vi "Get Indicator Data.vi"(6 "Connection ID":u64, 7 "Evaluate Pane Move":bool, 8 "error in (no error)":errorcluster, 9 "Values and Position":refnum<vi>[](array[refnum]), 10 "Get All":bool, 11 "Web FP In":refnum<class "Web Front Panel.lvclass">) -> (0 "error out":errorcluster, 2 "String":string, 3 "Web FP Out":refnum<class "Web Front Panel.lvclass">)   [LabVIEW 2017, in "Front Panel Publisher.lvlib" / "Web Front Panel.lvclass"]
uses:
  Web Front Panel.lvclass
  Front Panel Objects/Object_class/Object.lvclass
  Front Panel Publisher.lvlib
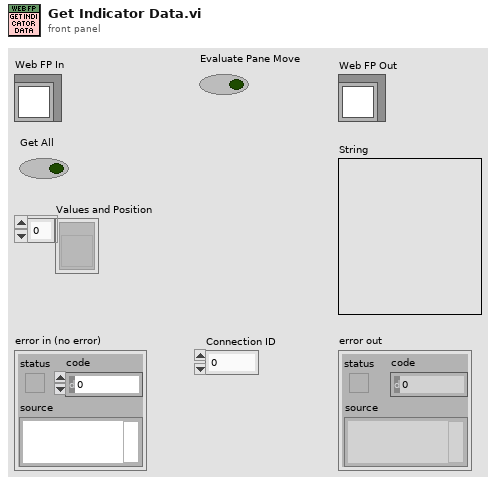
[diagram p1: front panel]
types:
  T1 = typedef "Front Panel Publisher.lvlib/Web Front Panel.lvclass/Object Attributes.ctl" = cluster{"VI Identifier":string, "VI Reference":refnum<vi>, "Controls":refnum<class "Object.lvclass">[], "Indicators":refnum<class "Object.lvclass">[], "Decorations":refnum<class "Object.lvclass">[], "VR With Previous Get":refnum<data-value>, "VR With Ring Images":refnum<data-value>}
  T2 = typedef "Front Panel Publisher.lvlib/Web Front Panel.lvclass/High Level Config Settings.ctl" = cluster{"Default Refresh Rate (ms)":i32, "Show Border":bool, "Periodic Decoration Data":bool, "Synchronous Requests":bool, "Reduce Sent Data":bool, "Recommended Control Settings":bool}
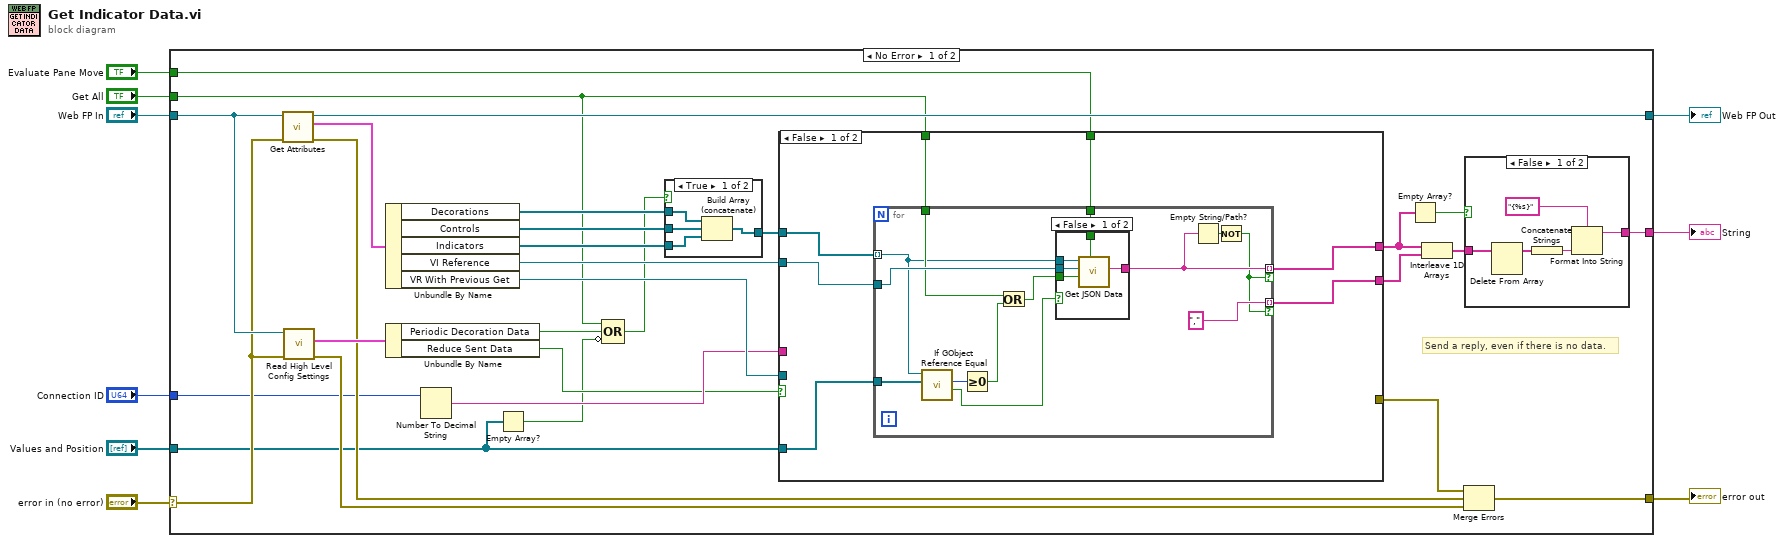
[diagram p0: block diagram]
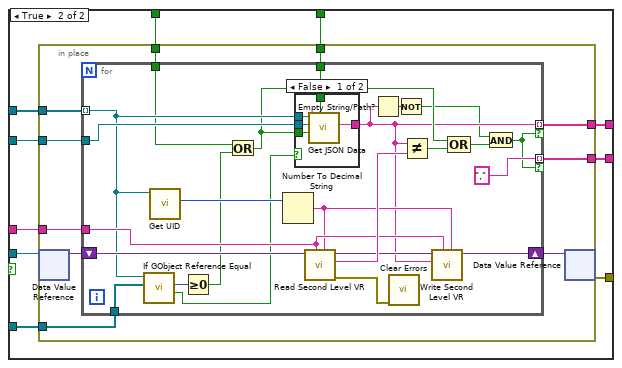
[diagram p3: hidden frame]
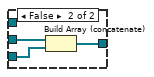
[diagram p5: hidden frame]
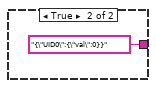
[diagram p6: hidden frame]
diagram:
  n1 = case shown="No Error" "error in (no error)" {
    selector: "error in (no error)" -> [w24 w127]
    tunnel: [w23 w127] -> w8
    tunnel: [w37 w126] -> w6
    tunnel: "Web FP In" -> [w25 w126]
    tunnel: [w33 _] -> w4
    tunnel: "Get All" -> [w14 _]
    tunnel: "Connection ID" -> [w18 _]
    tunnel: "Values and Position" -> [w15 _]
    tunnel: "Evaluate Pane Move" -> [w10 _]
    frame No Error {
      # "Send a reply, even if there is no data."
      n2 = call "Get Attributes.vi"("error in (no error)"=w24, "Web FP In"=w25) -> ("error out"=w21:errorcluster, "Data"=w38:T1, "Web FP Out"=w37:refnum<class "Web Front Panel.lvclass">)  [unwired: 6 in, 1 out]
      n3 = call "Read High Level Config Settings.vi"("error in (no error)"=w24, "Web FP In"=w25) -> ("error out"=w20:errorcluster, "High Level Config Settings"=w26:T2)  [unwired: 7 in, 1 out]
      n4 = Unbundle By Name(w38) -> ("Decorations"=w19:refnum<class "Object.lvclass">[], "Controls"=w30:refnum<class "Object.lvclass">[], "Indicators"=w32:refnum<class "Object.lvclass">[], "VI Reference"=w36:refnum<vi>, "VR With Previous Get"=w29:refnum<data-value>)
      n5 = Unbundle By Name(w26) -> ("Periodic Decoration Data"=w13:bool, "Reduce Sent Data"=w16:bool)
      n6 = Number To Decimal String(number=w18) -> (decimal integer string=w17:string)  [unwired: 1 in]
      n7 = Empty Array?(array=w15) -> (empty?=w12:bool)
      n8 = Compound Arithmetic op=OR(w14, w13, invert w12) -> (w11:bool)
      n9 = case shown="True" w11 {
        tunnel: w32 -> [w116 w119]
        tunnel: [w115 w118] -> w31
        tunnel: w30 -> [w114 w117]
        tunnel: w19 -> [w113 _]
        frame True {
          n10 = Build Array (concatenate)(w113, w114, w116) -> (w115:refnum<class "Object.lvclass">[])
        }
        frame False {
          n11 = Build Array (concatenate)(w117, w119) -> (w118:refnum<class "Object.lvclass">[])
        }
      }
      n12 = case shown="False" w16 {
        tunnel: w36 -> [w45 w73]
        tunnel: [w44 w72] -> w35
        tunnel: w31 -> [w43 w71]
        tunnel: w29 -> [_ w70]
        tunnel: [w42 w69] -> w28
        tunnel: w14 -> [w41 w68]
        tunnel: [_ w67] -> w22
        tunnel: w17 -> [_ w66]
        tunnel: w15 -> [w40 w65]
        tunnel: w10 -> [w39 w64]
        frame False {
          n13 = for {
            tunnel: w43 -> [w55] mode=indexing
            tunnel: w45 -> [w57]
            tunnel: [w51] -> w42 mode=indexing if=w49
            tunnel: [","] -> w44 mode=indexing if=w49
            tunnel: w41 -> [w56]
            tunnel: w40 -> [w54]
            tunnel: w39 -> [w46]
            n14 = call "If GObject Reference Equal.vi"("GObjects"=w54, "GObject in"=w55) -> ("Cluster Component"=w47:bool, "Index Found"=w53:i32)  [unwired: 6 in, 2 out]
            n15 = Greater Or Equal To 0?(x=w53) -> (x >= 0?=w52:bool)
            n16 = Or(x=w56, y=w52) -> (x .or. y?=w48:bool)
            n17 = case shown="False" w47 {
              tunnel: w57 -> [w63 _]
              tunnel: w55 -> [w62 _]
              tunnel: [w61 _] -> w51
              tunnel: w48 -> [w60 _]
              tunnel: w46 -> [w59 _]
              frame False {
                n18 = call-dynamic "Get JSON Data.vi"("Evaluate Pane Move"=w59, "Force Get All Data"=w60, "VI Reference"=w63, "Object In"=w62) -> ("JSON string"=w61:string)  [unwired: 5 in, 2 out]
              }
              frame True {
              }
            }
            n19 = Empty String/Path?(string/path=w51) -> (empty?=w50:bool)
            n20 = Not(x=w50) -> (.not. x?=w49:bool)
          }
        }
        frame True {
          n21 = in-place {
            in-place-border: w73 -> [w83]
            in-place-border: [w82] -> w69
            in-place-border: [w81] -> w72
            in-place-border: w71 -> [w80]
            in-place-border: w68 -> [w77]
            in-place-border: w66 -> [w76]
            in-place-border: w65 -> [w75]
            in-place-border: w64 -> [w74]
            n22 = in-place-dvr #1(w70) -> (w79:variant)  [unwired: 1 out]
            n23 = for {
              tunnel: w80 -> [w94] mode=indexing
              tunnel: w83 -> [w106]
              tunnel: [w88] -> w82 mode=indexing if=w87
              tunnel: [","] -> w81 mode=indexing if=w87
              shift-right: [w96] -> w78
              shift-left: w79 -> [w102]
              tunnel: w77 -> [w91]
              tunnel: w76 -> [w98]
              tunnel: w75 -> [w93]
              tunnel: w74 -> [w84]
              n24 = call "If GObject Reference Equal.vi"("GObjects"=w93, "GObject in"=w94) -> ("Cluster Component"=w85:bool, "Index Found"=w95:i32)  [unwired: 6 in, 2 out]
              n25 = call-dynamic "Get UID.vi"("Object In"=w94) -> ("UID"=w105:i32)  [unwired: 8 in, 2 out]
              n26 = Greater Or Equal To 0?(x=w95) -> (x >= 0?=w92:bool)
              n27 = Or(x=w91, y=w92) -> (x .or. y?=w90:bool)
              n28 = Number To Decimal String(number=w105) -> (decimal integer string=w97:string)  [unwired: 1 in]
              n29 = case shown="False" w85 {
                tunnel: w106 -> [w112 _]
                tunnel: w94 -> [w111 _]
                tunnel: w90 -> [w110 _]
                tunnel: [w109 _] -> w88
                tunnel: w84 -> [w108 _]
                frame False {
                  n30 = call-dynamic "Get JSON Data.vi"("Evaluate Pane Move"=w108, "Force Get All Data"=w110, "VI Reference"=w112, "Object In"=w111) -> ("JSON string"=w109:string)  [unwired: 5 in, 2 out]
                }
                frame True {
                }
              }
              n31 = call "Read Second Level VR.vi"("Tag"=w97, "Section"=w98, "Variant Repository In"=w102) -> ("error out"=w101:errorcluster, "Value"=w100:string, "Variant Repository Out"=w99:variant)  [unwired: 6 in]
              n32 = Empty String/Path?(string/path=w88) -> (empty?=w89:bool)
              n33 = call <vilib>:"Clear Errors.vi"("error in (no error)"=w101) -> ()  [unwired: 5 in, 2 out]
              n34 = Not(x=w89) -> (.not. x?=w86:bool)
              n35 = Not Equal?(x=w88, y=w100) -> (x != y?=w104:bool)
              n36 = call "Write Second Level VR.vi"("Tag"=w97, "Section"=w98, "Value"=w88, "Variant Repository In"=w99) -> ("Variant Repository Out"=w96:variant)  [unwired: 6 in, 1 out]
              n37 = Compound Arithmetic op=OR(w90, w104) -> (w103:bool)
              n38 = And(x=w86, y=w103) -> (x .and. y?=w87:bool)
            }
            n39 = in-place-dvr #1(w78) -> (w67:errorcluster)  [unwired: 1 out]
          }
        }
      }
      n40 = Empty Array?(array=w28) -> (empty?=w27:bool)
      n41 = Interleave 1D Arrays(w28, w35) -> (w34:string[])
      n42 = Merge Errors(w22, w21, w20) -> (w23:errorcluster)
      n43 = case shown="False" w27 {
        tunnel: w34 -> [w124 _]
        tunnel: [w120 "{\"UID0\":{\"val\":0}}"] -> w33
        frame False {
          n44 = Delete From Array(array=w124) -> (array with subset deleted=w123:string[])  [unwired: 2 in, 1 out]
          n45 = Concatenate Strings(w123) -> (w122:string)
          n46 = Format Into String(format string="{%s}", w122) -> (resulting string=w120:string)  [unwired: 2 in, 1 out]
        }
        frame True {
        }
      }
    }
    frame Error {
    }
  }
  "error out" <- w8
  "Web FP Out" <- w6
  "String" <- w4
